vi "Test Latch when released.vi"(11 "Error in":errorcluster) -> (15 "Error out":errorcluster)   [LabVIEW 2020, in "Mechanical Actions Tests.lvlib"]
doc: "This VI is used to test latch when released function"
uses:
  Mechanical Actions Tests.lvlib
  <vilib>/addons/_JKI Toolkits/Caraya/classes/Test Suite/Define Test Suite (JUnit Report).vi
  <vilib>/SLL Drona/APIs/Stimulus/ControlValue/SetValueAuto.vi
  <vilib>/SLL Drona/APIs/Assert/AssertControlValue/Equal.vi
  <vilib>/SLL Drona/APIs/Stimulus/VI/CloseVI.vi
  <vilib>/Utility/error.llb/Error Cluster From Error Code.vi
  <vilib>/ErrorRing/Error Ring.xnode
  <vilib>/addons/_JKI Toolkits/Caraya/classes/Test Suite/Test Suite.lvclass
  <vilib>/SLL Drona/Drona.lvlib
  <vilib>/SLL Drona/APIs/Stimulus/ControlValue/ControlValue.lvlib
  <vilib>/SLL Drona/APIs/Assert/AssertControlValue/AssertControlValue.lvlib
  <vilib>/addons/_JKI Toolkits/Caraya/classes/Test/Test.lvclass
  <vilib>/Wiresmith Technology/G CLI/CLI Class/CLI.lvclass
  <vilib>/SLL Drona/APIs/Stimulus/VI/VI.lvlib
panel:
  # "LATCH WHEN RELEASED TEST"
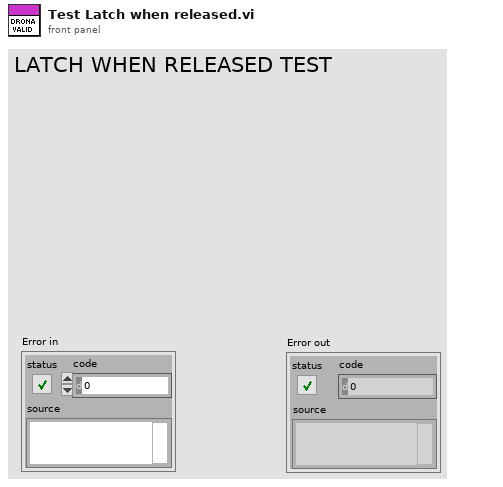
[diagram p1: front panel]
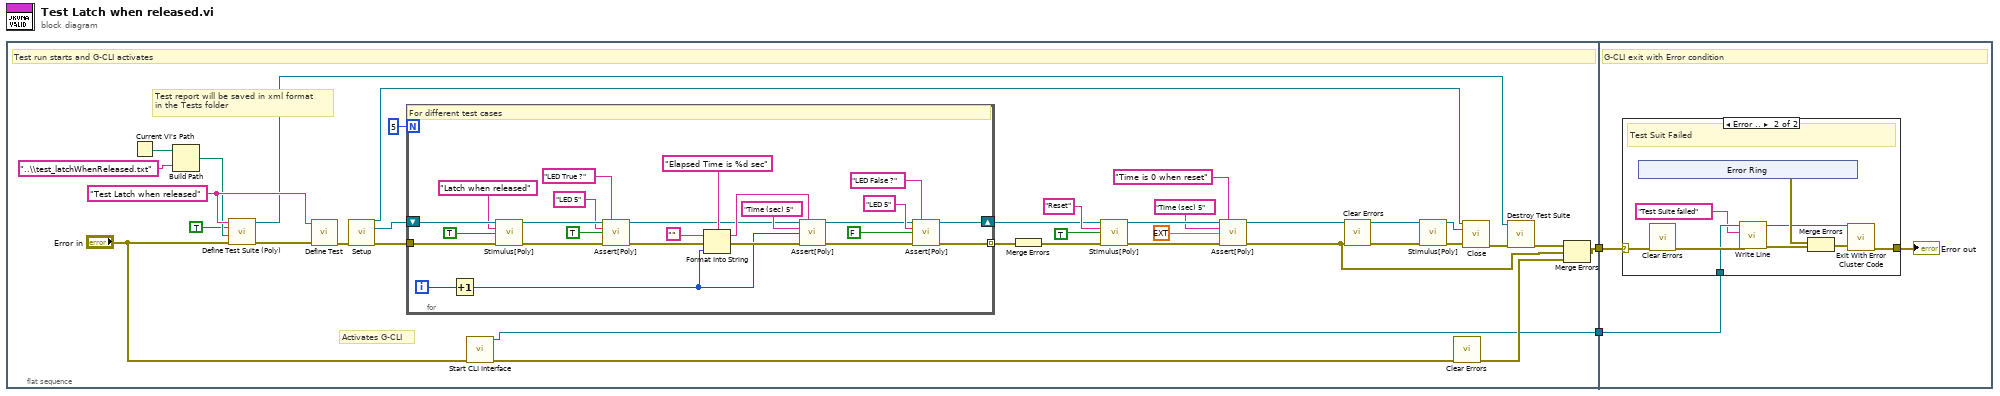
[diagram p0: block diagram]
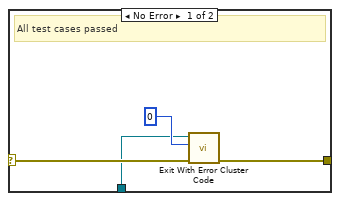
[diagram p2: hidden frame]
diagram:
  n1 = flat-sequence {
    tunnel: [w5] -> w2
    tunnel: [w17] -> w1
    tunnel: w2 -> [w64]
    tunnel: w1 -> [w63]
    frame #0 {
      w15 = "Test Latch when released" ("Label (VI Title)")
      # "Test report will be saved in xml format\nin the Tests folder"
      # "Activates G-CLI"
      # "Test run starts and G-CLI activates"
      n2 = Current VI's Path() -> (path=w13:path)
      n3 = Build Path(base path=w13, name or relative path="..\\test_latchWhenReleased.txt") -> (appended path=w11:path)
      n4 = call-poly <vilib>:"Define Test Suite (Poly).vi"("error in (no error)"="Error in", "Report Path"=w11, "Interactive"=TRUE, "Label (VI Title)"=w15) -> ("error out"=w16:errorcluster, "Test Suite"=w7:refnum<class "Test Suite.lvclass">)  [unwired: 5 in, 1 out]
      n5 = call <vilib>:"Define Test.vi"("error in (no error)"=w16, "Label (VI Title)"=w15) -> ("error out"=w36:errorcluster)  [unwired: 8 in, 1 out]
      n6 = call <vilib>:"Setup.vi"("error in"=w36) -> ("Application Ref"=w25:refnum<vi>, "VI Reference Out"=w35:refnum<vi>, "error out"=w23:errorcluster)  [unwired: 12 in]
      n7 = for {
        N: 5 -> [_]
        shift-right: [w42] -> w27
        shift-left: w35 -> [w60]
        tunnel: w23 -> [w61]
        tunnel: [w43] -> w26 mode=indexing
        i -> [w53]
        # "For different test cases"
        n8 = Increment(x=w53) -> (x+1=w49:i32)
        n9 = call-poly <vilib>:"Stimulus[Poly].vi"("VI Reference In"=w60, "Control Path"="Latch when released", "Value (Signaling)"=TRUE, "error in"=w61) -> ("VI Reference Out"=w46:refnum<vi>, "error out"=w47:errorcluster)  [unwired: 10 in]
        n10 = call-poly <vilib>:"Assert[Poly].vi"("VI Reference In"=w46, "Test Label"="LED True ?" ("Label"), "Control Path"="LED 5", "Control Value"=TRUE, "Error In"=w47) -> ("VI Reference Out"=w37:refnum<vi>, "Error Out"=w38:errorcluster)  [unwired: 9 in]
        n11 = Format Into String(format string="Elapsed Time is %d sec", initial string="", error in=w38, w49) -> (resulting string=w48:string, error out=w52:errorcluster)
        n12 = call-poly <vilib>:"Assert[Poly].vi"("VI Reference In"=w37, "Test Label"=w48, "Control Path"="Time (sec) 5", "Control Value"=w49, "Error In"=w52) -> ("VI Reference Out"=w45:refnum<vi>, "Error Out"=w44:errorcluster)  [unwired: 9 in]
        n13 = call-poly <vilib>:"Assert[Poly].vi"("VI Reference In"=w45, "Test Label"="LED False ?" ("Label"), "Control Path"="LED 5", "Control Value"=FALSE, "Error In"=w44) -> ("VI Reference Out"=w42:refnum<vi>, "Error Out"=w43:errorcluster)  [unwired: 9 in]
      }
      n14 = call <vilib>:"Start CLI Interface.vi"("error in (no error)"="Error in") -> ("error out"=w6:errorcluster, "CLI out"=w5:refnum<class "CLI.lvclass">)  [unwired: 7 in, 2 out]
      n15 = Merge Errors(w26) -> (w24:errorcluster)
      n16 = call-poly <vilib>:"Stimulus[Poly].vi"("VI Reference In"=w27, "Control Path"="Reset", "Value (Signaling)"=TRUE, "error in"=w24) -> ("VI Reference Out"=w34:refnum<vi>, "error out"=w33:errorcluster)  [unwired: 10 in]
      n17 = call-poly <vilib>:"Assert[Poly].vi"("VI Reference In"=w34, "Test Label"="Time is 0 when reset" ("Label"), "Control Path"="Time (sec) 5", "Control Value"=ext 0.0, "Error In"=w33) -> ("VI Reference Out"=w21:refnum<vi>, "Error Out"=w3:errorcluster)  [unwired: 9 in]
      n18 = call <vilib>:"Clear Errors.vi"("error in (no error)"=w3) -> ("error out"=w4:errorcluster)  [unwired: 5 in, 1 out]
      n19 = call-poly <vilib>:"Stimulus[Poly].vi"("VI Reference In"=w21, "error in"=w4) -> ("VI Reference Out"=w20:refnum<vi>, "error out"=w19:errorcluster)  [unwired: 12 in]
      n20 = call <vilib>:"Clear Errors.vi"("error in (no error)"=w6) -> ("error out"=w18:errorcluster)  [unwired: 5 in, 1 out]
      n21 = call <vilib>:"Close.vi"("Application Ref"=w25, "VI Reference"=w20, "error in"=w19) -> ("error out"=w8:errorcluster)  [unwired: 12 in]
      n22 = call-dynamic "Destroy Test Suite.vi"("error in (no error)"=w8, "Test Suite in"=w7) -> ("error out"=w9:errorcluster)  [unwired: 8 in, 1 out]
      n23 = Merge Errors(w9, w3, w18) -> (w17:errorcluster)
    }
    frame #1 {
      # "G-CLI exit with Error condition"
      n24 = case shown="Error .." w63 {
        selector: w63 -> [w68 w76]
        tunnel: w64 -> [w65 w74]
        tunnel: [w67 w77] -> w62
        frame No Error {
          # "All test cases passed"
          n25 = call <vilib>:"Exit With Error Cluster Code.vi"("error in (no error)"=w68, "No Error Code (0)"=0, "CLI in"=w65) -> ("error out"=w67:errorcluster)  [unwired: 8 in]
        }
        frame Error {
          # "Test Suit Failed"
          n26 = xnode "Error Ring"() -> ("error out"=w71:errorcluster)
          n27 = call <vilib>:"Clear Errors.vi"("error in (no error)"=w76) -> ("error out"=w75:errorcluster)  [unwired: 5 in, 1 out]
          n28 = call <vilib>:"Write Line.vi"("error in (no error)"=w75, "Text to Write"="Test Suite failed", "CLI in"=w74) -> ("error out"=w70:errorcluster, "CLI out"=w69:refnum<class "CLI.lvclass">)  [unwired: 7 in]
          n29 = Merge Errors(w71, w70) -> (w72:errorcluster)
          n30 = call <vilib>:"Exit With Error Cluster Code.vi"("error in (no error)"=w72, "CLI in"=w69) -> ("error out"=w77:errorcluster)  [unwired: 9 in]
        }
      }
      "Error out" <- w62
    }
  }
